vi "TSM Sync Pins to Sessions.vi"(0 "TSM context":T2, 5 "Pins":tag[](array[tag]), 11 "error in":errorcluster) -> (4 "TSM Sync Out":T1, 15 "error out":errorcluster)   [LabVIEW 2020]
doc: "Populates the TSM Sync cluster for the specified pin(s) and pin group(s)."
uses:
  <vilib>/NI_TestStand_SemiconductorModule/NI_TestStand_Semiconductor_Module.lvlibp/PinMap/General/SemiconductorModuleContext.ctl
  TSM Sync.ctl
  <vilib>/NI_TestStand_SemiconductorModule/NI_TestStand_Semiconductor_Module.lvlibp/PinMap/PinQueryContext/MultiplePinMultipleSessionQueryContext/MultiplePinMultipleSessionQueryContext.lvclass
  <vilib>/NI_TestStand_SemiconductorModule/NI_TestStand_Semiconductor_Module.lvlibp
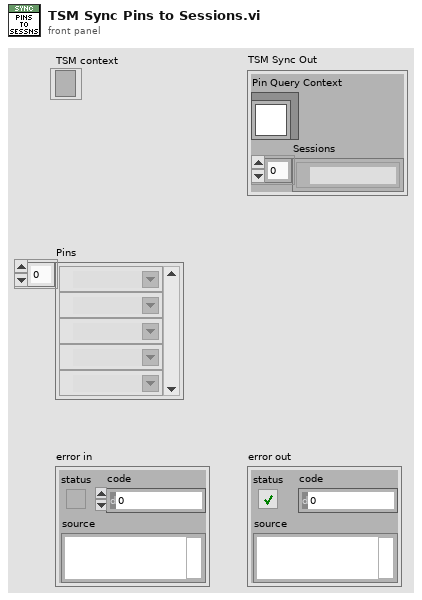
[diagram p1: front panel]
types:
  T1 = typedef "TSM Sync.ctl" = cluster{"Pin Query Context":refnum<class "MultiplePinMultipleSessionQueryContext.lvclass">, "Sessions":refnum<k15>[]}
  T2 = typedef "NI_TestStand_Semiconductor_Module.lvlibp/SemiconductorModuleContext.ctl" = refnum<k7>
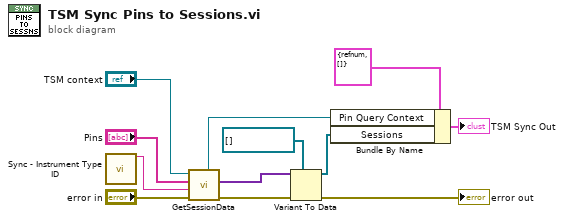
[diagram p0: block diagram]
diagram:
  n1 = call "Sync - Instrument Type ID.vi"() -> ("Instrument Type ID"=w6:string)  [unwired: 15 in]
  n2 = call <vilib>:"GetSessionData.vi"("error in (no error)"="error in", "Instrument Type Id"=w6, "Pins"="Pins", "Semiconductor Module Context"="TSM context") -> ("error out"=w9:errorcluster, "Session Data"=w10:variant[], "Pin Query Context"=w2:refnum<class "MultiplePinMultipleSessionQueryContext.lvclass">)  [unwired: 2 in, 3 out]
  n3 = Variant To Data(error in=w9, type=refnum<k15>[] [] ("Instrument Sessions"), Variant=w10) -> (data=w3:refnum<k15>[], error out=→"error out":errorcluster)
  n4 = Bundle By Name(cluster=T1 {"Pin Query Context"=refnum, "Sessions"=[]} ("TSM Sync Out"), "Pin Query Context"=w2, "Sessions"=w3) -> (→"TSM Sync Out":T1)
